vi "VectorNav-ReadYPR.vi"() -> ()   [LabVIEW 2010]
uses:
  <vilib>/Instr/_visa.llb/VISA Configure Serial Port (Instr).vi
panel:
  out "read buffer":string
  in  "stop":bool
  out "Roll":dbl
  out "Pitch":dbl
  out "Heading":dbl
  in  "VISA resource name":refnum<visa-resource-name>="COM1"
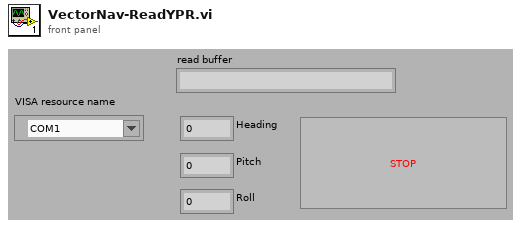
[diagram p1: front panel]
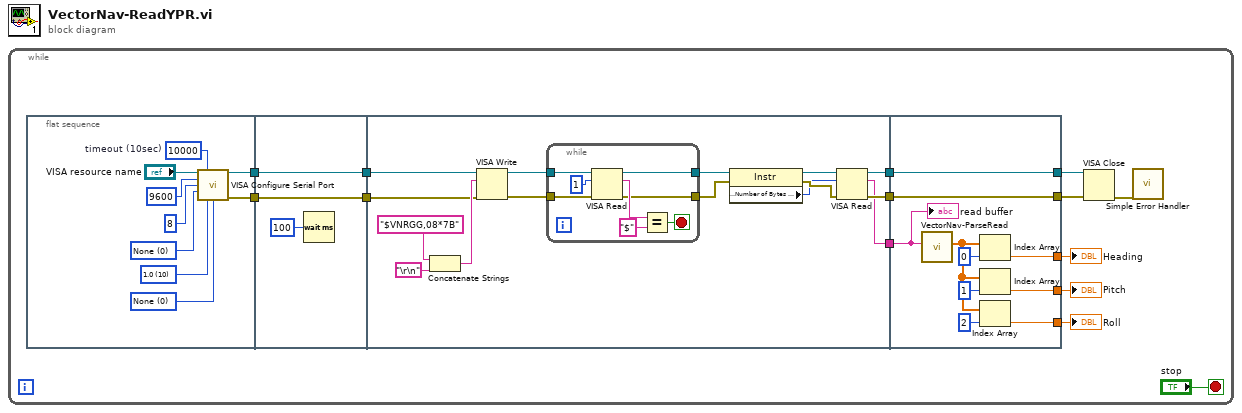
[diagram p0: block diagram]
diagram:
  n1 = while {
    stop <- "stop" stop-if-true
    n2 = flat-sequence {
      tunnel: [w15] -> w14
      tunnel: [w16] -> w13
      tunnel: w14 -> [w25]
      tunnel: w13 -> [w24]
      tunnel: [w25] -> w11
      tunnel: [w24] -> w12
      tunnel: [w34] -> w10
      tunnel: [w33] -> w9
      tunnel: [w32] -> w8
      tunnel: w12 -> [w28]
      tunnel: w11 -> [w27]
      tunnel: [w58] -> w5
      tunnel: [w59] -> w6
      tunnel: w10 -> [w59]
      tunnel: w9 -> [w58]
      tunnel: w8 -> [w57]
      tunnel: [w56] -> w4
      tunnel: [w52] -> w3
      tunnel: [w51] -> w2
      frame #0 {
        w18 = u16 0 items=["None"=0, "XON/XOFF"=1, "RTS/CTS"=2, "DTR/DSR"=4] ("flow control")
        w19 = u16 10 items=["1.0"=10, "1.5"=15, "2.0"=20] ("stop bits")
        w21 = u16 0 items=["None", "Odd", "Even", "Mark", "Space"] ("parity")
        w20 = u32 10000  # timeout (10sec)
        n3 = call-poly "VISA Configure Serial Port"("VISA resource name"="VISA resource name", "timeout (10sec)"=w20, "baud rate (9600)"=u32 9600 ("baud rate"), "data bits (8)"=u16 8 ("data bits"), "parity (0:none)"=w21, "stop bits (10: 1 bit)"=w19, "flow control (0:none)"=w18) -> ("VISA resource name out"=w16:refnum<visa-resource-name>, "error out"=w15:errorcluster)  [unwired: 2 in, 5 out]
      }
      frame #1 {
        n4 = Wait (ms)(milliseconds to wait=u32 100) -> ()  [unwired: 1 out]
      }
      frame #2 {
        n5 = Concatenate Strings("$VNRGG,08*7B" ("string"), "\r\n") -> (w29:string)
        n6 = VISA Write(VISA resource name=w28, write buffer=w29, error in (no error)=w27) -> (VISA resource name out=w36:refnum<visa-resource-name>, error out=w35:errorcluster)  [unwired: 1 out]
        n7 = while {
          tunnel: [w45] -> w37
          tunnel: [w44] -> w38
          tunnel: w36 -> [w43]
          tunnel: w35 -> [w42]
          stop <- w46 stop-if-true
          n8 = VISA Read(VISA resource name=w43, byte count=u32 1, error in (no error)=w42) -> (VISA resource name out=w45:refnum<visa-resource-name>, read buffer=w48:string, error out=w44:errorcluster)  [unwired: 1 out]
          n9 = Equal?(x=w48, y="$") -> (x = y?=w46:bool)
        }
        n10 = property class="Instr"(reference=w37, error in=w38) -> (reference out=w40:refnum<visa-resource-name>, error out=w41:errorcluster, "Serial Settings:Number of Bytes at Serial Port"=w39:u32)
        n11 = VISA Read(VISA resource name=w40, byte count=w39, error in (no error)=w41) -> (VISA resource name out=w34:refnum<visa-resource-name>, read buffer=w32:string, error out=w33:errorcluster)  [unwired: 1 out]
      }
      frame #3 {
        n12 = call "VectorNav-ParseRead.vi"("Input String"=w57) -> ("Output Array"=w55:dbl[])  [unwired: 10 in]
        n13 = Index Array(array=w55, index=0) -> (element=w56:dbl)
        n14 = Index Array(array=w55, index=1) -> (element=w52:dbl)
        n15 = Index Array(array=w55, index=2) -> (element=w51:dbl)
        "read buffer" <- w57
      }
    }
    n16 = VISA Close(VISA resource name=w6, error in (no error)=w5) -> (error out=w7:errorcluster)
    n17 = call <vilib>:"Simple Error Handler.vi"("error in (no error)"=w7) -> ()  [unwired: 1 in, 8 out]
    "Heading" <- w4
    "Pitch" <- w3
    "Roll" <- w2
  }
